vi "Limit Switch Saftey Handle.vi"(1 "Lower Limit":bool, 2 "Motor In":dbl, 3 "Upper Limit":bool) -> (0 "Motor Out":dbl)   [LabVIEW 2017]
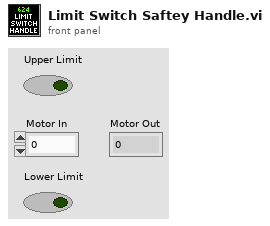
[diagram p1: front panel]
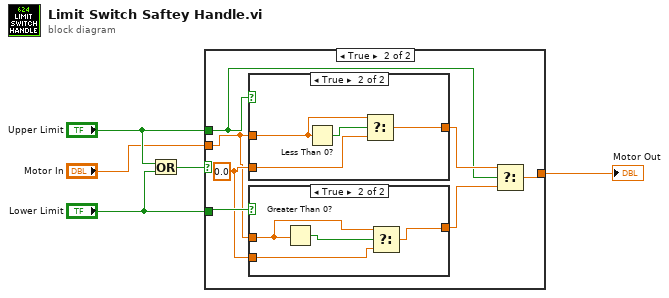
[diagram p0: block diagram]
diagram:
  n1 = Or(x="Upper Limit", y="Lower Limit") -> (x .or. y?=w5:bool)
  n2 = case shown="True" w5 {
    tunnel: "Upper Limit" -> [_ w7]
    tunnel: "Lower Limit" -> [_ w13]
    tunnel: "Motor In" -> [w6 w11]
    tunnel: [w6 w10] -> w1
    frame False {
    }
    frame True {
      w12 = 0.0
      n3 = case shown="True" w7 {
        tunnel: w12 -> [_ w22]
        tunnel: w11 -> [w19 w21]
        tunnel: [w19 w20] -> w9
        frame False {
        }
        frame True {
          n4 = Less Than 0?(x=w21) -> (x < 0?=w23:bool)
          n5 = Select(t=w21, s=w23, f=w22) -> (s? t:f=w20:dbl)
        }
      }
      n6 = case shown="True" w13 {
        tunnel: w12 -> [_ w17]
        tunnel: w11 -> [w14 w16]
        tunnel: [w14 w15] -> w8
        frame False {
        }
        frame True {
          n7 = Greater Than 0?(x=w16) -> (x > 0?=w18:bool)
          n8 = Select(t=w16, s=w18, f=w17) -> (s? t:f=w15:dbl)
        }
      }
      n9 = Select(t=w9, s=w7, f=w8) -> (s? t:f=w10:dbl)
    }
  }
  "Motor Out" <- w1
